vi "Sample Main VI 2.vi"(11 "Input":dbl) -> (3 "Output":dbl)   [LabVIEW 2019]
doc: "This VI is used to demonstrate the addition of a VI to a project."
panel:
  # "Sample Main VI 2"
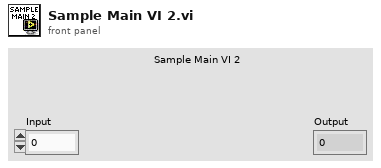
[diagram p1: front panel]
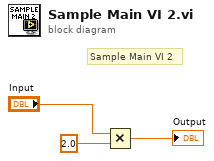
[diagram p0: block diagram]
diagram:
  # "Sample Main VI 2"
  n1 = Multiply(x="Input", y=2.0) -> (x*y=→"Output":dbl)
